vi "Autonomous Independent.vi"   [LabVIEW 2015]
doc: "This VI is called when autonomous begins, and will automatically be terminated when autonomous ends. You can carry out timed or sensor driven robot movement independently without needing to return to the caller."
panel:
  # "Be sure to right-click and choose Data Operations>>Make Current Value default if you want to save the array values with the VI"
types:
  T1 = typedef "WPI_MotorControlDeviceRef.ctl" = cluster{"DeviceStatus":errorcluster, "Type":T2, "PWM":cluster{"PWM Channel":T3, "DeadBand":T4}, "CAN":cluster{"Device Number":u8, "Control Mode":T5, "Semaphore":T6, "Max Vout":dbl, "TalonSRX Control Mode":T7}, "Invert":bool}
  T2 = typedef "WPI_MotorControlType.ctl" = enum16{"PWM", "CAN", "CANTalonSRX"}
  T3 = typedef "FPGA_DIOPWMChannel.ctl" = enum8{"PWM 0", "PWM 1", "PWM 2", "PWM 3", "PWM 4", "PWM 5", "PWM 6", "PWM 7", "PWM 8", "PWM 9", "PWM MXP 0", "PWM MXP 1", "PWM MXP 2", "PWM MXP 3", "PWM MXP 4", "PWM MXP 5", "PWM MXP 6", "PWM MXP 7", "PWM MXP 8", "PWM MXP 9", "Invalid"}
  T4 = typedef "WPI_PWMDeadband.ctl" = cluster{"Name":string, "maxPositivePwm":i32, "minPositivePwm":i32, "centerPwm":i32, "maxNegativePwm":i32, "minNegativePwm":i32, "angularRange":u16}
  T5 = typedef "WPI_CANJaguar_ControlMode.ctl" = enum8{"Percent VBus", "Current", "Speed", "Position", "Voltage"}
  T6 = typedef "Semaphore RefNum" = refnum<k1>
  T7 = typedef "WPI_CANTalonSRX_APIControlMode.ctl" = enum8{"Percent VBus", "Speed", "Position", "Slave", "Unchanged / Invalid", "Voltage Compensation", "Current", "Motion Profile"}
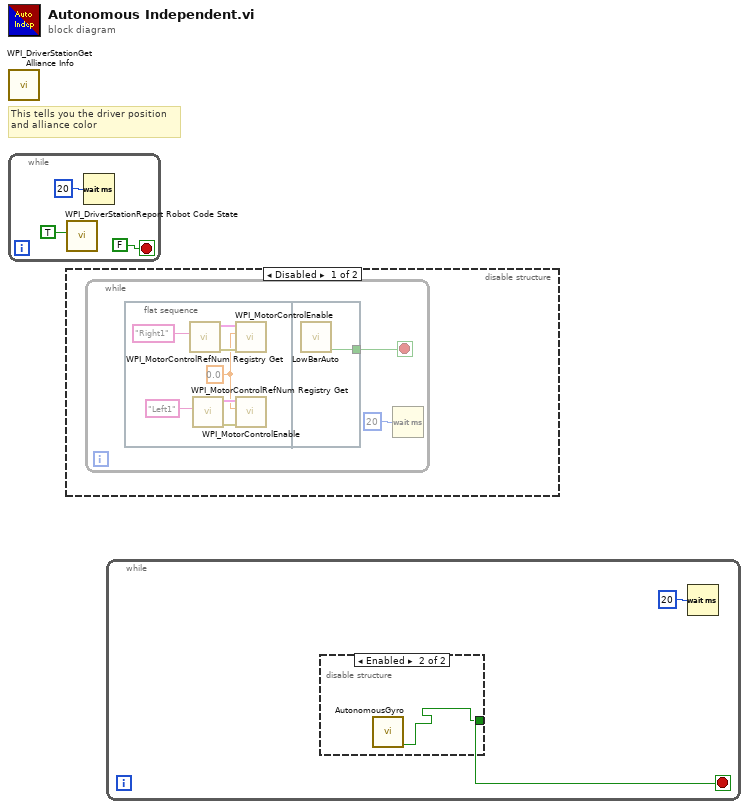
[diagram p0: block diagram]
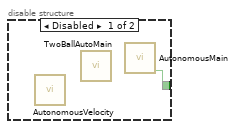
[diagram p2: hidden frame]
diagram:
  # "This tells you the driver position\nand alliance color"
  n1 = call <vilib>:"WPI_DriverStationGet Alliance Info.vi"() -> ()  [unwired: 12 out]
  n2 = while {
    stop <- FALSE stop-if-true
    n3 = call <vilib>:"WPI_DriverStationReport Robot Code State.vi"("Autonomous"=TRUE) -> ()  [unwired: 10 in, 1 out]
    n4 = Wait (ms)(milliseconds to wait=u32 20) -> ()  [unwired: 1 out]
  }
  n5 = disable-structure shown="Disabled" {
    frame Disabled {
      n6 = while {
        stop <- w5 stop-if-true
        n7 = flat-sequence {
          tunnel: [w13] -> w5
          frame #0 {
            w6 = 0.0 ("Encoder Initial Position")
            n8 = call <vilib>:"WPI_MotorControlRefNum Registry Get.vi"("refnum name"="Right1") -> ("error out"=w9:errorcluster, "MotorControlDevRef"=w10:T1)  [unwired: 9 in]
            n9 = call <vilib>:"WPI_MotorControlRefNum Registry Get.vi"("refnum name"="Left1") -> ("error out"=w7:errorcluster, "MotorControlDevRef"=w8:T1)  [unwired: 9 in]
            n10 = call <vilib>:"WPI_MotorControlEnable.vi"("error in (no error)"=w9, "Encoder Initial Position"=w6, "CAN MotorDevRef"=w10) -> ()  [unwired: 7 in, 2 out]
            n11 = call <vilib>:"WPI_MotorControlEnable.vi"("error in (no error)"=w7, "Encoder Initial Position"=w6, "CAN MotorDevRef"=w8) -> ()  [unwired: 7 in, 2 out]
          }
          frame #1 {
            n12 = call "LowBarAuto.vi"() -> ("Terminate"=w13:bool)  [unwired: 11 in]
          }
        }
        n13 = Wait (ms)(milliseconds to wait=u32 20) -> ()  [unwired: 1 out]
      }
    }
    frame Enabled {
    }
  }
  n14 = while {
    stop <- w14 stop-if-true
    n15 = disable-structure shown="Enabled" {
      disable-tunnel: [w16 w17] -> w14
      frame Disabled {
        n16 = call "AutonomousVelocity.vi"() -> ()  [unwired: 11 in, 1 out]
        n17 = call "TwoBallAutoMain.vi"() -> ()  [unwired: 12 in]
        n18 = call "AutonomousMain.vi"() -> ("Terminate"=w16:bool)  [unwired: 11 in]
      }
      frame Enabled {
        n19 = call "AutonomousGyro.vi"() -> ("Terminate"=w17:bool)  [unwired: 11 in]
      }
    }
    n20 = Wait (ms)(milliseconds to wait=u32 20) -> ()  [unwired: 1 out]
  }
